vi "Read UID.vi"(8 "error in (no error)":errorcluster, 11 "GObject in":refnum<class "GObject.lvclass">) -> (0 "error out":errorcluster, 2 "UID":i32, 3 "GObject out":refnum<class "GObject.lvclass">)   [LabVIEW 2023, in "TLC_Scripto.lvlib" / "GObject.lvclass"]
uses:
  GObject.lvclass
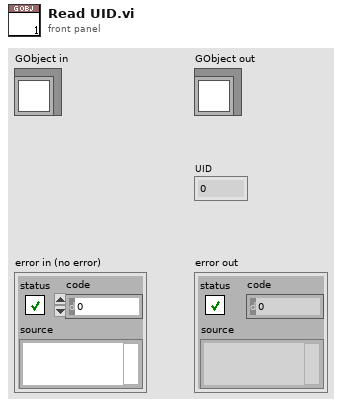
[diagram p1: front panel]
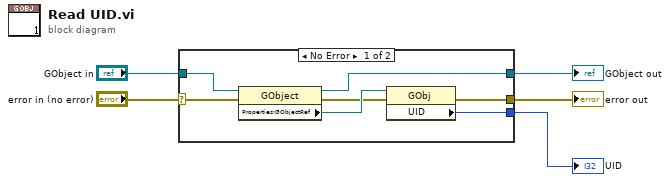
[diagram p0: block diagram]
diagram:
  n1 = case shown="No Error" "error in (no error)" {
    selector: "error in (no error)" -> [w9 w14]
    tunnel: [w12 w14] -> w4
    tunnel: [w7 w13] -> w2
    tunnel: "GObject in" -> [w6 w13]
    tunnel: [w11 _] -> w1
    frame No Error {
      n2 = property class="GObject"(reference=w6, error in=w9) -> (reference out=w7:refnum<class "GObject.lvclass">, error out=w8:errorcluster, "Properties:GObjectRef"=w10:refnum<vi>)
      n3 = property class="GObj"(reference=w10, error in=w8) -> (error out=w12:errorcluster, "UID"=w11:i32)  [unwired: 1 out]
    }
    frame Error {
    }
  }
  "error out" <- w4
  "GObject out" <- w2
  "UID" <- w1
